vi "motor query error status.vi"(8 "error in (no error)":errorcluster, 11 "Handle In":i32) -> (0 "error out":errorcluster, 2 "Error state":bool=TRUE, 3 "Handle Out":i32)   [LabVIEW 2013]
uses:
  motor constants.ctl
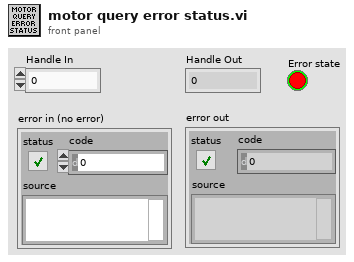
[diagram p1: front panel]
types:
  T1 = typedef "motor constants.ctl" = u16
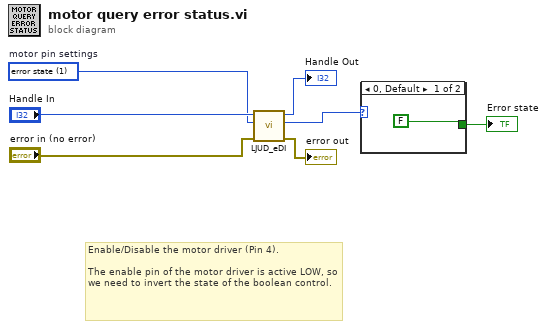
[diagram p0: block diagram]
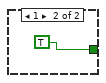
[diagram p2: hidden frame]
diagram:
  w3 = T1 1 items=["reset"=0, "error state"=1, "enable"=4, "direction"=5, "step"=6, "end switch"=7]  # motor pin settings
  # "Enable/Disable the motor driver (Pin 4).\n\nThe enable pin of the motor driver is active LOW, so we need to invert the state of the boolean control."
  n1 = call <vilib>:"LJUD_eDI.vi"("error in"="error in (no error)", "Channel"=w3, "Handle In"="Handle In") -> ("error out"=→"error out":errorcluster, "State"=w1:i32, "Handle Out"=→"Handle Out":i32)  [unwired: 6 in]
  n2 = case shown="0, Default" w1 {
    tunnel: [FALSE ("Error state 2") TRUE ("Error state 2")] -> w2
    frame 0, Default {
    }
    frame 1 {
    }
  }
  "Error state" <- w2
